vi "LOG Update PID.vi"(10 "data":variant, 11 "key":string) -> ()   [LabVIEW 2019, in "Log.lvlib"]
uses:
  Log.lvlib
  SubVIs/Shared/System GV.vi
  SubVIs/Shared/Shared.lvlib
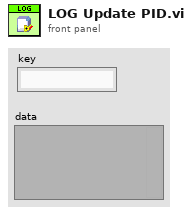
[diagram p1: front panel]
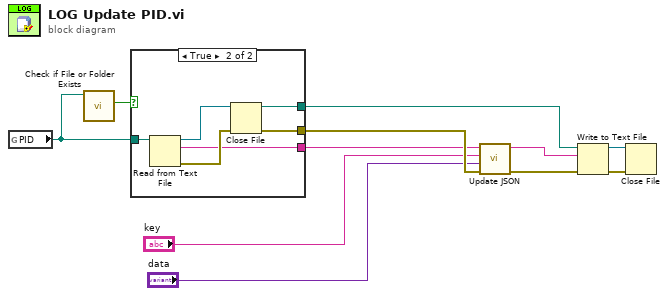
[diagram p0: block diagram]
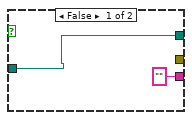
[diagram p2: hidden frame]
diagram:
  n1 = global read "System GV.vi" "PID"() -> (w10:path)
  n2 = call <vilib>:"Check if File or Folder Exists.vi"("path"=w10) -> ("file or folder exists?"=w1:bool)  [unwired: 8 in, 2 out]
  n3 = case shown="True" w1 {
    tunnel: [_ w19] -> w11
    tunnel: w10 -> [w13 w18]
    tunnel: [w13 w17] -> w3
    tunnel: ["" w14] -> w2
    frame False {
    }
    frame True {
      n4 = Read from Text File(file (use dialog)=w18) -> (refnum out=w15:refnum<file>, text=w14:string, error out=w16:errorcluster)  [unwired: 3 in, 1 out]
      n5 = Close File(refnum=w15, error in=w16) -> (path=w17:path, error out=w19:errorcluster)
    }
  }
  n6 = call "Update JSON.vi"("error in (no error)"=w11, "Value"="data", "key"="key", "JSON in"=w2) -> ("error out"=w7:errorcluster, "JSON out"=w4:string)  [unwired: 6 in]
  n7 = Write to Text File(file (use dialog)=w3, text=w4, error in=w7) -> (refnum out=w6:refnum<file>, error out=w5:errorcluster)  [unwired: 1 in, 1 out]
  n8 = Close File(refnum=w6, error in=w5) -> ()  [unwired: 2 out]
